vi "Acquisition Message Loop.vi"(8 "error in (no error)":errorcluster, 9 "Data Queue":refnum<queue>, 10 "Data Notifier":refnum<notifier>, 11 "Message Queues":T1) -> (0 "error out":errorcluster)   [LabVIEW 2013, in "Acquisition.lvlib"]
doc: "Message loop for handling messages pertaining to the acquisition of data from the hardware."
uses:
  Acquisition.lvlib
  support/Message Queue/All Message Queues.ctl
  support/Message Queue/Message Cluster.ctl
  Hardware Configuration.ctl
  Signal Type.ctl
  Acquisition State.ctl
  controls/UI Data.ctl
  <vilib>/Utility/error.llb/DialogType.ctl
  <vilib>/Utility/error.llb/Error Cluster From Error Code.vi
  support/Message Queue/Enqueue Message (Single).vi
  <vilib>/ErrorRing/Error Ring.xnode
  support/Message Queue/Message Queue.lvlib
  support/Message Queue/Enqueue Message (MultiLine String w Array).vi
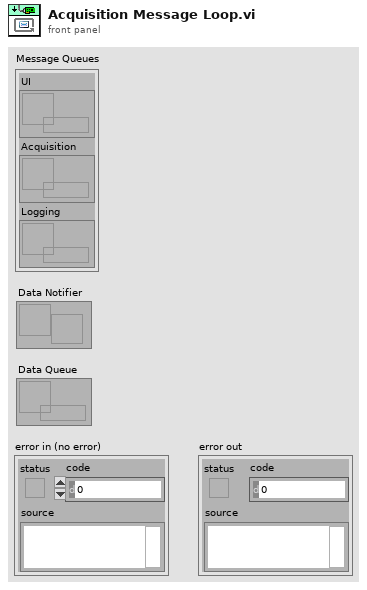
[diagram p1: front panel]
types:
  T1 = typedef "Message Queue.lvlib/All Message Queues.ctl" = cluster{"UI":refnum<queue>, "Acquisition":refnum<queue>, "Logging":refnum<queue>}
  T2 = cluster{"Macro:Initialize":string, "Macro:Exit":string, "Core":cluster{"Current VI Reference":refnum<vi>, "Close Panel on Exit?":bool}}
  T3 = typedef "UI Data.ctl" = cluster{"Start Ref":refnum<vi>, "Stop Ref":refnum<vi>, "Settings Ref":refnum<vi>, "Exit Ref":refnum<vi>, "Status Ref":refnum<vi>, "Data Ref":refnum<vi>}
  T4 = typedef "Acquisition.lvlib/Acquisition State.ctl" = enum16{"Idle", "Acquiring"}
  T5 = typedef "Acquisition.lvlib/Hardware Configuration.ctl" = cluster{"HW Refnum <Replace Me>":string, "Signal Type <Replace Me>":T6}
  T6 = typedef "Acquisition.lvlib/Signal Type.ctl" = enum16{"Sine Wave", "Square with Noise"}
  T7 = enum32{"invalid app kind", "Development System", "Run Time System", "Student Edition", "Embedded LabVIEW", "Evaluation", "Custom"}
  T8 = enum32{"Invalid", "Standard", "Closed", "Hidden", "Minimized", "Maximized"}
  T9 = typedef "DialogType.ctl" = u16
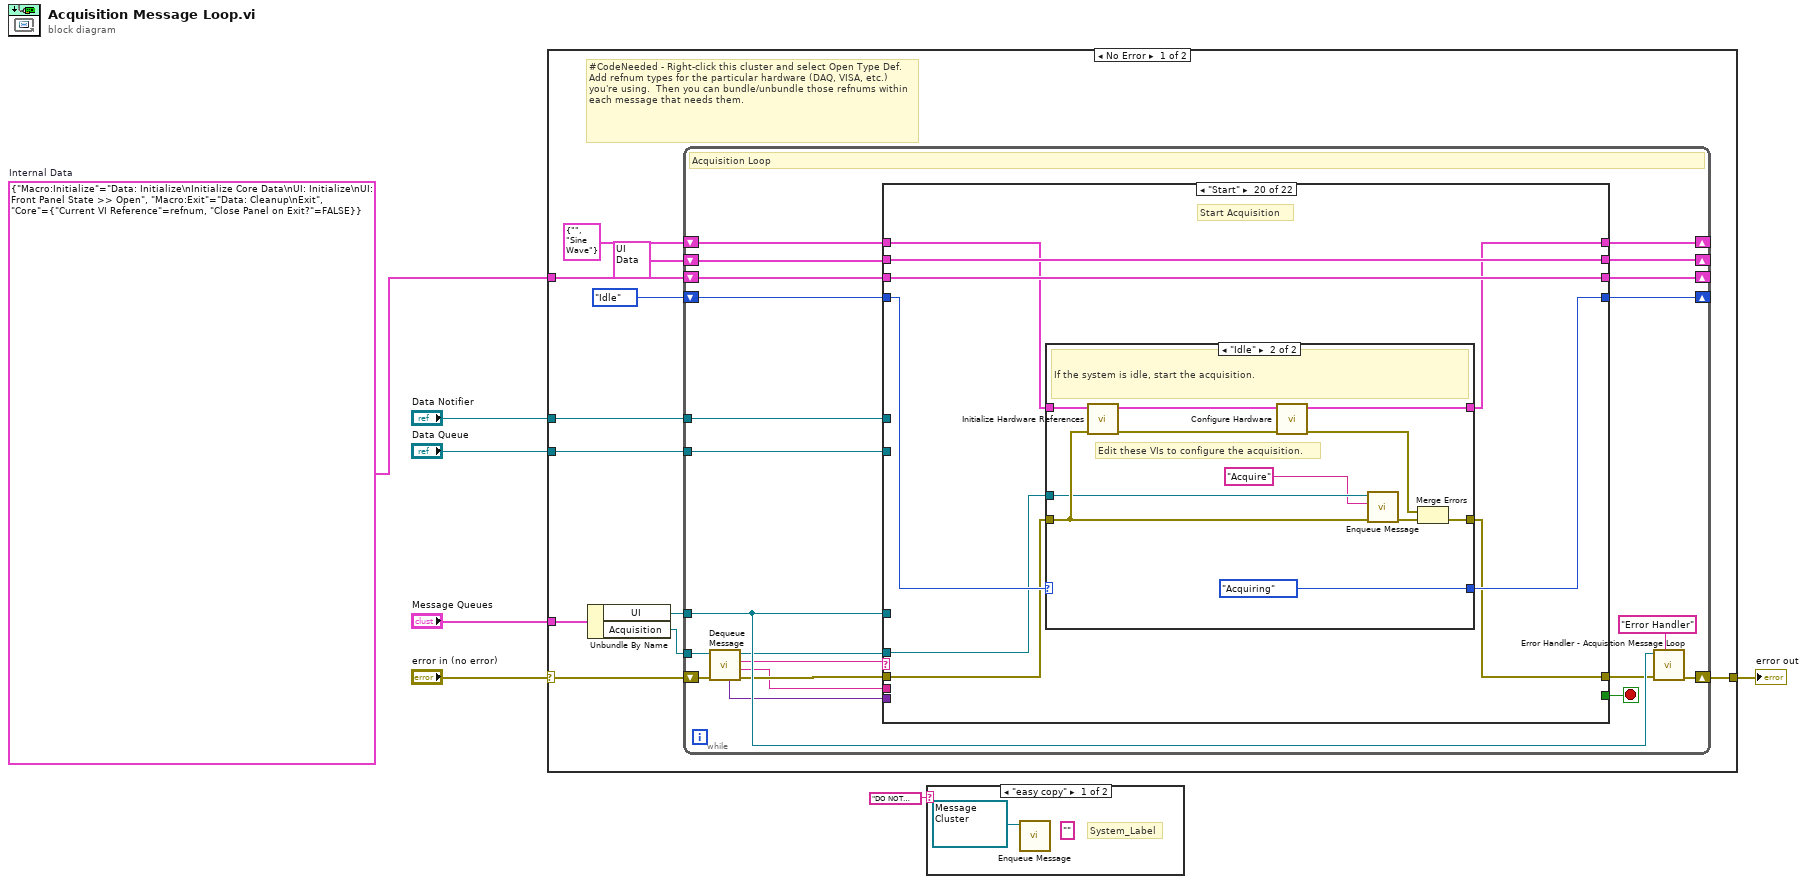
[diagram p0: block diagram]
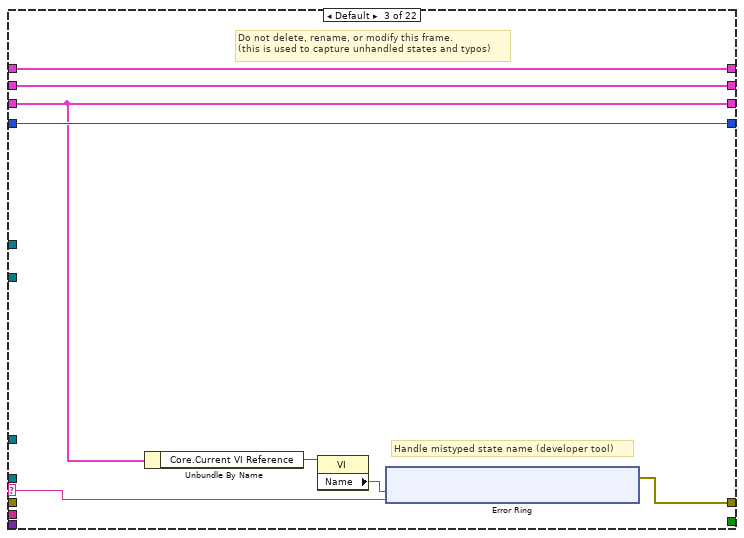
[diagram p5: hidden frame]
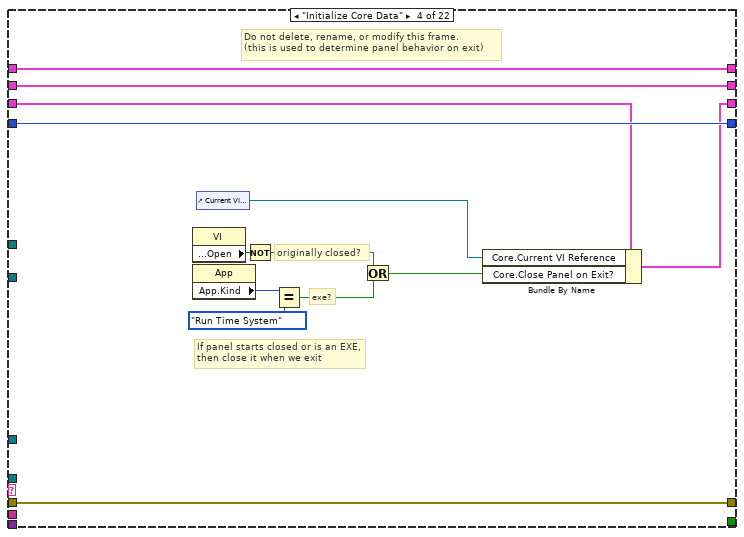
[diagram p6: hidden frame]
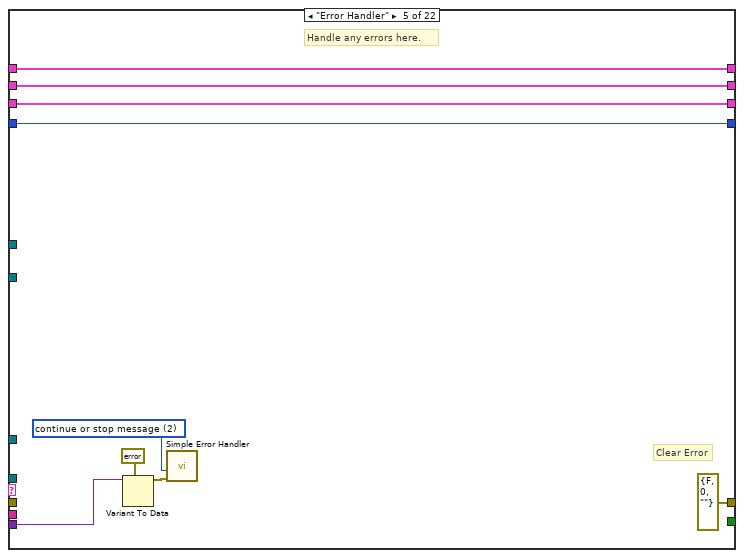
[diagram p7: hidden frame]
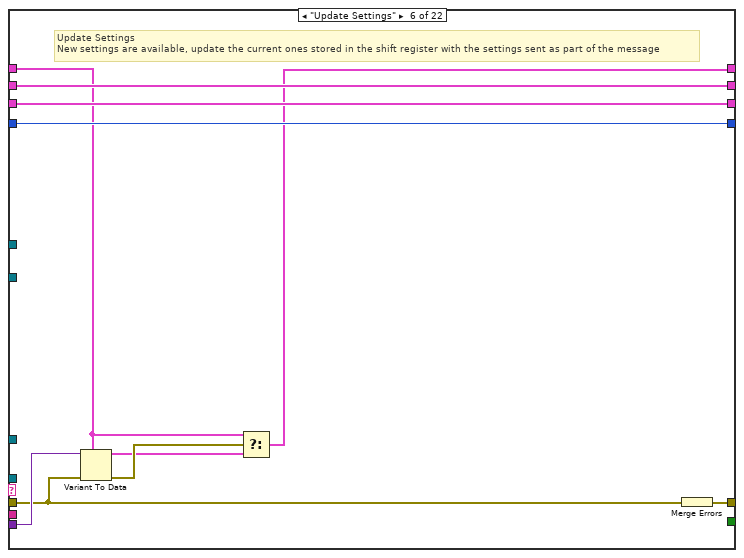
[diagram p8: hidden frame]
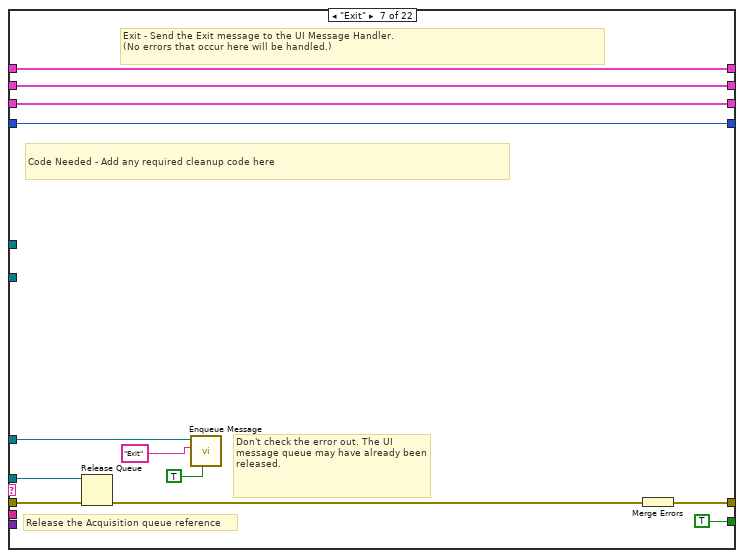
[diagram p9: hidden frame]
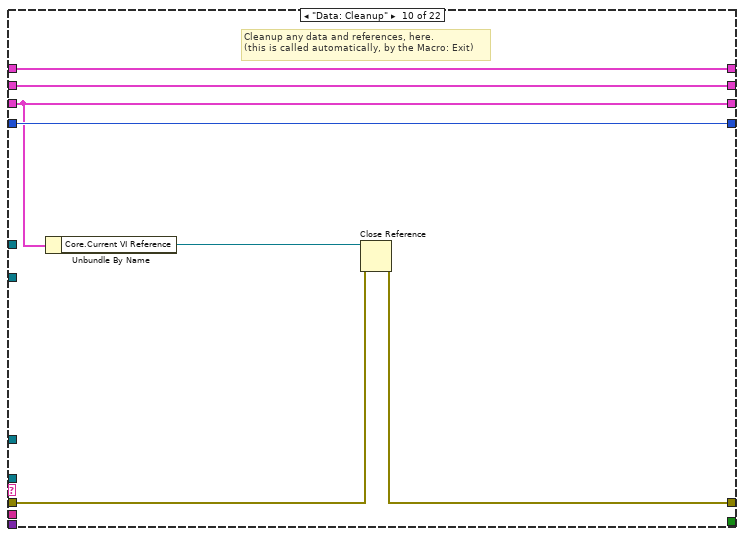
[diagram p12: hidden frame]
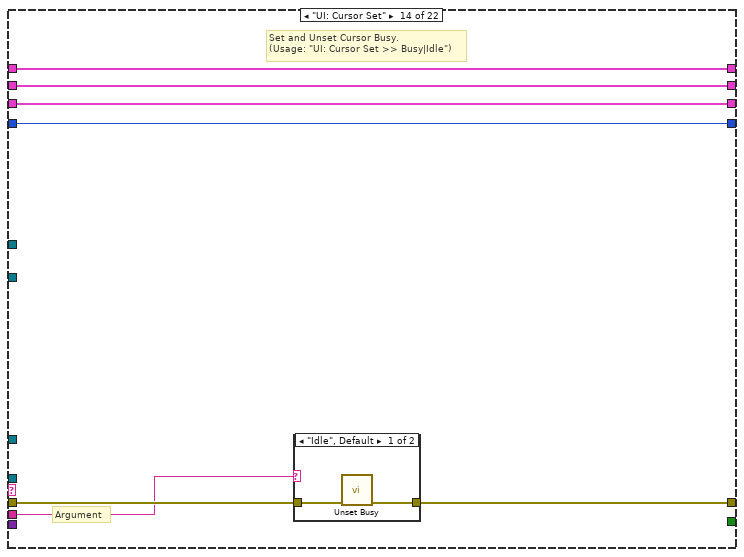
[diagram p16: hidden frame]
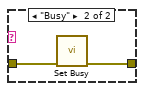
[diagram p17: hidden frame]
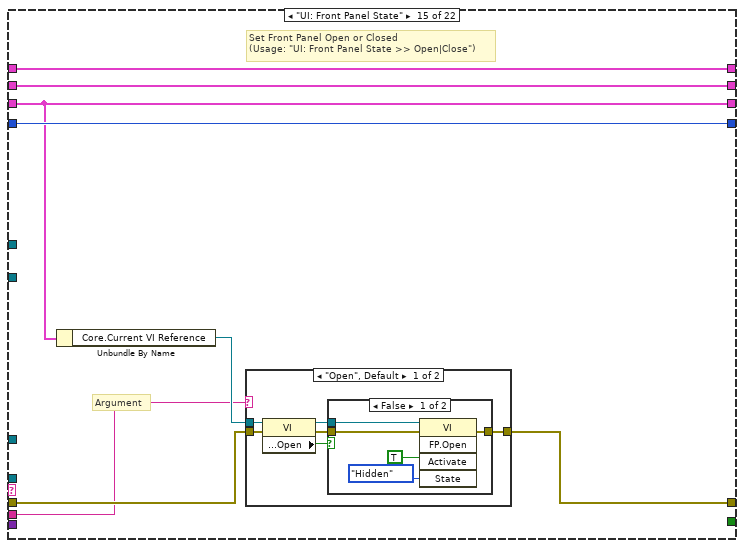
[diagram p18: hidden frame]
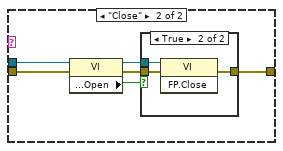
[diagram p20: hidden frame]
diagram:
  w2 = T2 {"Macro:Initialize"="Data: Initialize\nInitialize Core Data\nUI: Initialize\nUI: Front Panel State >> Open", "Macro:Exit"="Data: Cleanup\nExit", "Core"={"Current VI Reference"=refnum, "Close Panel on Exit?"=FALSE}}  # Internal Data
  n1 = case shown="No Error" "error in (no error)" {
    selector: "error in (no error)" -> [w14 w284]
    tunnel: "Message Queues" -> [w18 _]
    tunnel: [w16 w284] -> w6
    tunnel: "Data Notifier" -> [w12 _]
    tunnel: "Data Queue" -> [w11 _]
    tunnel: w2 -> [w9 _]
    frame No Error {
      # "#CodeNeeded - Right-click this cluster and select Open Type Def.  Add refnum types for the particular hardware (DAQ, VISA, etc.) you're using.  Then you can bundle/unbundle those refnums within each message that needs them."
      n2 = Unbundle By Name(w18) -> ("UI"=w13:refnum<queue>, "Acquisition"=w17:refnum<queue>)
      n3 = while {
        tunnel: w17 -> [w39]
        shift-right: [w22] -> _
        shift-left: T5 {"HW Refnum <Replace Me>"="", "Signal Type <Replace Me>"=enum."Sine Wave"} ("Data Cluster") -> [w29]
        shift-right: [w38] -> w16
        shift-left: w14 -> [w40]
        tunnel: w13 -> [w37]
        tunnel: w12 -> [w21]
        tunnel: w11 -> [w20]
        shift-right: [w23] -> _
        shift-left: Acquisition_State."Idle" ("State") -> [w27]
        shift-right: [w25] -> _
        shift-left: T3 {"Start Ref"=refnum, "Stop Ref"=refnum, "Settings Ref"=refnum, "Exit Ref"=refnum, "Status Ref"=refnum, "Data Ref"=refnum} ("Measurement UI Controls") -> [w26]
        shift-right: [w24] -> _
        shift-left: w9 -> [w28]
        stop <- w36 stop-if-true
        # "Acquisition Loop"
        n4 = call "Dequeue Message.vi"("error in (no error)"=w40, "Message Queue"=w39) -> ("error out"=w32:errorcluster, "Argument"=w31:string, "Message"=w33:string, "dup Message Queue"=w34:refnum<queue>, "Message Data"=w30:variant)  [unwired: 5 in]
        n5 = case shown="\"Start\"" w33 {
          selector: w33 -> [_ _ w53 _ _ _ _ _ _ _ _ _ _ _ _ _ _ _ _ _ w241 _]
          tunnel: w26 -> [w44 w48 w57 w71 w88 w98 w108 w113 w120 w123 w130 w135 w140 w145 w156 w186 w195 w209 w215 w226 w252 w274]
          tunnel: w31 -> [_ _ _ _ _ _ _ _ _ _ _ _ _ w146 w157 _ _ _ _ _ _ _]
          tunnel: w29 -> [w43 w49 w58 w69 w86 w92 w110 w114 w116 w124 w131 w137 w142 w149 w159 w187 w196 w207 w216 w219 w250 w268]
          tunnel: [w45 w50 w51 w79 errorcluster {"status"=FALSE, "code"=0, "source"=""} ("error out") w90 w100 w115 w117 w125 w132 w136 w141 w147 w160 w188 w191 w197 w217 w221 w242 w267] -> w35
          tunnel: w32 -> [w45 w50 _ w79 _ w89 w105 w115 w117 w126 w132 w136 w141 w148 w161 w188 w193 w206 w217 w222 w243 w270]
          tunnel: [w44 w48 w57 w71 w88 w98 w108 w113 w120 w123 w130 w135 w140 w145 w156 w186 w195 w209 w215 w226 w252 w274] -> w25
          tunnel: [_ _ _ _ _ _ TRUE _ _ _ _ _ _ _ _ _ _ _ _ _ _ _] -> w36
          tunnel: [w43 w49 w58 w69 w86 w91 w110 w114 w116 w124 w131 w137 w142 w149 w159 w187 w196 w207 w216 w218 w249 w268] -> w22
          tunnel: [w42 w47 w56 w70 w87 w97 w107 w112 w119 w122 w129 w134 w139 w144 w155 w185 w194 w208 w214 w223 w247 w271] -> w23
          tunnel: w27 -> [w42 w47 w56 w70 w87 w97 w107 w112 w119 w122 w129 w134 w139 w144 w155 w185 w194 w208 w214 w224 w248 w272]
          tunnel: w30 -> [_ _ _ _ w82 w95 _ _ _ _ _ _ _ _ _ _ _ _ _ _ _ _]
          tunnel: w28 -> [w41 w46 w52 w68 w85 w96 w106 w111 w118 w121 w128 w133 w138 w143 w154 w184 w189 w200 w213 w225 w251 w273]
          tunnel: [w41 w46 w52 w67 w85 w96 w106 w111 w118 w121 w128 w133 w138 w143 w154 w184 w189 w200 w213 w225 w251 w273] -> w24
          tunnel: w34 -> [_ _ _ _ _ _ w104 _ _ _ _ _ _ _ _ _ w192 w205 _ w220 w244 _]
          tunnel: w37 -> [_ _ _ _ _ _ w103 _ _ _ _ _ _ _ _ _ _ _ _ _ _ w269]
          tunnel: w21 -> [_ _ _ _ _ _ _ _ _ _ _ _ _ _ _ _ _ _ _ _ w246 _]
          tunnel: w20 -> [_ _ _ _ _ _ _ _ _ _ _ _ _ _ _ _ _ _ _ _ w245 _]
          frame "", "Idle" {
            # "Executes when the state queue is empty\nAlso commented out messages"
          }
          frame "---------- Core ----------" {
            # "Do not put any code in this frame.\n(it is a separator no-op)"
          }
          frame Default {
            # "Handle mistyped state name (developer tool)"
            # "Do not delete, rename, or modify this frame.\n(this is used to capture unhandled states and typos)"
            n6 = Unbundle By Name(w52) -> ("Core.Current VI Reference"=w54:refnum<vi>)
            n7 = property class="VI"(reference=w54) -> ("Name"=w55:string)  [unwired: 1 in, 2 out]
            n8 = xnode "Error Ring"("parameter 0"=w55, "parameter 1"=w53) -> ("error out"=w51:errorcluster)
          }
          frame "Initialize Core Data" {
            # "Do not delete, rename, or modify this frame.\n(this is used to determine panel behavior on exit)"
            # "originally closed?"
            # "exe?"
            # "If panel starts closed or is an EXE, then close it when we exit"
            n9 = property class="VI"() -> ("Front Panel.Open"=w78:bool)  [unwired: 2 in, 2 out]
            n10 = property class="App"() -> ("App.Kind"=w77:T7)  [unwired: 2 in, 2 out]
            n11 = control-ref of="Current VI Reference"() -> (w72:refnum<vi>)
            n12 = Not(x=w78) -> (.not. x?=w75:bool)
            n13 = Equal?(x=w77, y=T7."Run Time System" ("Application:Kind")) -> (x = y?=w74:bool)
            n14 = Or(x=w75, y=w74) -> (x .or. y?=w73:bool)
            n15 = Bundle By Name(cluster=w68, "Core.Current VI Reference"=w72, "Core.Close Panel on Exit?"=w73) -> (w67:T2)
          }
          frame "Error Handler" {
            w81 = T9 2 items=["no dialog", "OK message", "continue or stop message", "OK message + warnings", "continue/stop + warnings"] ("type of dialog (OK msg:1)")
            # "Clear Error"
            # "Handle any errors here."
            n16 = Variant To Data(type=errorcluster {"status"=FALSE, "code"=0, "source"=""} ("error constant"), Variant=w82) -> (data=w84:errorcluster)  [unwired: 1 in, 1 out]
            n17 = call <vilib>:"Simple Error Handler.vi"("type of dialog (OK msg:1)"=w81, "error in (no error)"=w84) -> ()  [unwired: 3 in, 5 out]
          }
          frame "Update Settings" {
            # "Update Settings\nNew settings are available, update the current ones stored in the shift register with the settings sent as part of the message"
            n18 = Variant To Data(error in=w89, type=w92, Variant=w95) -> (data=w93:T5, error out=w94:errorcluster)
            n19 = Select(t=w92, s=w94, f=w93) -> (s? t:f=w91:T5)
            n20 = Merge Errors(w89) -> (w90:errorcluster)
          }
          frame "Exit" {
            # "Code Needed - Add any required cleanup code here"
            # "Exit - Send the Exit message to the UI Message Handler.\n(No errors that occur here will be handled.)"
            # "Don't check the error out. The UI message queue may have already been released."
            # "Release the Acquisition queue reference"
            n21 = Release Queue(queue=w104, error in (no error)=w105) -> (error out=w99:errorcluster)  [unwired: 1 in, 2 out]
            n22 = call-poly "Enqueue Message.vi"("Priority Message? (F)"=TRUE, "Message"="Exit", "Message Queue"=w103) -> ()  [unwired: 7 in, 2 out]
            n23 = Merge Errors(w99) -> (w100:errorcluster)
          }
          frame "---------- Data ----------" {
            # "Do not put any code in this frame.\n(It is a separator no-op. You can make a copy of this frame to create a new Data frame)"
          }
          frame "Data: Initialize" {
            # "nothing right now"
            # "Initialize the shift-register data, here.\n(data names are defined by what you wire into the bundle function)"
          }
          frame "Data: Cleanup" {
            # "Cleanup any data and references, here.\n(this is called automatically, by the Macro: Exit)"
            n24 = Unbundle By Name(w121) -> ("Core.Current VI Reference"=w127:refnum<vi>)
            n25 = Close Reference(reference=w127, error in (no error)=w126) -> (error out=w125:errorcluster)
          }
          frame "---------- UI ----------" {
            # "Do not put any code in this frame.\n(It is a separator no-op. You can make a copy of this frame to create a new UI frame)"
          }
          frame "UI: Initialize" {
            # "Initialize the User Interface, here.\n(this is called automatically, by the Macro: Init)"
          }
          frame "UI: Initialize UI Refs" {
            # "Package and Init UI Refs as Required"
          }
          frame "UI: Cursor Set" {
            # "Argument"
            # "Set and Unset Cursor Busy.\n(Usage: \"UI: Cursor Set >> Busy|Idle\")"
            n26 = case shown="\"Idle\", Default" w146 {
              tunnel: w148 -> [w151 w153]
              tunnel: [w150 w152] -> w147
              frame "Idle", Default {
                n27 = call <vilib>:"Unset Busy.vi"("error in (no error)"=w151) -> ("error out"=w150:errorcluster)  [unwired: 10 in]
              }
              frame "Busy" {
                n28 = call <vilib>:"Set Busy.vi"("error in (no error)"=w153) -> ("error out"=w152:errorcluster)  [unwired: 9 in, 1 out]
              }
            }
          }
          frame "UI: Front Panel State" {
            # "Argument"
            # "Set Front Panel Open or Closed\n(Usage: \"UI: Front Panel State >> Open|Close\")"
            n29 = Unbundle By Name(w154) -> ("Core.Current VI Reference"=w158:refnum<vi>)
            n30 = case shown="\"Open\", Default" w157 {
              tunnel: w161 -> [w165 w178]
              tunnel: [w167 w179] -> w160
              tunnel: w158 -> [w166 w176]
              frame "Open", Default {
                n31 = property class="VI"(reference=w166, error in=w165) -> (reference out=w163:refnum<vi>, error out=w164:errorcluster, "Front Panel.Open"=w162:bool)
                n32 = case shown="False" w162 {
                  tunnel: [w170 w173] -> w167
                  tunnel: w164 -> [w169 w173]
                  tunnel: w163 -> [w168 _]
                  frame False {
                    n33 = invoke class="VI" method="FP.Open"(reference=w168, error in=w169, "Activate"=TRUE, "State"=T8."Hidden") -> (error out=w170:errorcluster)  [unwired: 1 in, 4 out]
                  }
                  frame True {
                  }
                }
              }
              frame "Close" {
                n34 = property class="VI"(reference=w176, error in=w178) -> (reference out=w175:refnum<vi>, error out=w177:errorcluster, "Front Panel.Open"=w174:bool)
                n35 = case shown="True" w174 {
                  tunnel: [w180 w183] -> w179
                  tunnel: w177 -> [w180 w182]
                  tunnel: w175 -> [_ w181]
                  frame False {
                  }
                  frame True {
                    n36 = invoke class="VI" method="FP.Close"(reference=w181, error in=w182) -> (error out=w183:errorcluster)  [unwired: 1 in, 2 out]
                  }
                }
              }
            }
          }
          frame "---------- Macro ----------" {
            # "Do not put any code in this frame.\n(It is a separator no-op. You can make a copy of this frame to create a new Macro frame)"
          }
          frame "Macro: Initialize" {
            # "Initialization Macro\n(This is called once, when the VI starts)"
            n37 = Unbundle By Name(w189) -> ("Macro:Initialize"=w190:string)
            n38 = call-poly "Enqueue Message.vi"("error in (no error)"=w193, "Message"=w190, "Message Queue"=w192) -> ("error out"=w191:errorcluster)  [unwired: 7 in, 1 out]
          }
          frame "Macro: Exit" {
            # "Exit Macro\n(This is called once, when the VI exits)"
            n39 = Unbundle By Name(w200) -> ("Core.Close Panel on Exit?"=w212:bool)
            n40 = Unbundle By Name(w200) -> ("Macro:Exit"=w199:string)
            n41 = Select(t="UI: Front Panel State >> Close", s=w212, f="") -> (s? t:f=w204:string)
            n42 = call-poly "Enqueue Message.vi"("Priority Message? (F)"=TRUE, "error in (no error)"=w206, "Message"=w204, "Message Queue"=w205) -> ("error out"=w201:errorcluster, "dup Message Queue"=w202:refnum<queue>)  [unwired: 6 in]
            n43 = call-poly "Enqueue Message.vi"("Priority Message? (F)"=FALSE, "error in (no error)"=w201, "Message"=w199, "Message Queue"=w202) -> ("error out"=w197:errorcluster)  [unwired: 6 in, 1 out]
          }
          frame "---------- Acquisition ----------" {
            # "Acquisition Section"
          }
          frame "Start" {
            # "Start Acquisition"
            n44 = case shown="\"Idle\"" w224 {
              selector: w224 -> [w227 _]
              tunnel: [w228 w240] -> w221
              tunnel: w219 -> [w229 w239]
              tunnel: w222 -> [w228 w238]
              tunnel: w220 -> [_ w236]
              tunnel: [w229 w232] -> w218
              tunnel: [w227 Acquisition_State."Acquiring" ("Acquisition State")] -> w223
              frame "Acquiring" {
                # "The system is already acquiring. Ignore the \"Start\" message."
              }
              frame "Idle" {
                # "Edit these VIs to configure the acquisition."
                # "If the system is idle, start the acquisition."
                n45 = call "Initialize Hardware References.vi"("error in (no error)"=w238, "Hardware Resources in"=w239) -> ("error out"=w235:errorcluster, "Hardware Resources out"=w233:T5)  [unwired: 8 in]
                n46 = call "Configure Hardware.vi"("error in (no error)"=w235, "Hardware Resources in"=w233) -> ("error out"=w234:errorcluster, "Hardware Resources out"=w232:T5)  [unwired: 8 in]
                n47 = call-poly "Enqueue Message.vi"("error in (no error)"=w238, "Message"="Acquire", "Message Queue"=w236) -> ("error out"=w237:errorcluster)  [unwired: 7 in, 1 out]
                n48 = Merge Errors(w234, w237) -> (w240:errorcluster)
              }
            }
          }
          frame "Acquire" {
            # "Acquire Data"
            n49 = case shown="\"Acquiring\"" w248 {
              selector: w248 -> [w253 w258]
              tunnel: [w254 w266] -> w242
              tunnel: w244 -> [_ w264]
              tunnel: w243 -> [w254 w257]
              tunnel: [w255 w262] -> w249
              tunnel: w250 -> [w255 w261]
              tunnel: w246 -> [_ w260]
              tunnel: w245 -> [_ w259]
              tunnel: [w253 w258] -> w247
              tunnel: w241 -> [_ w256]
              frame "Idle" {
                # "Ignore \"Acquire\" messages when the acquisition is idle."
              }
              frame "Acquiring" {
                # "Acquire more data while in the \"Acquiring\" state."
                n50 = call "Acquire.vi"("error in (no error)"=w257, "Data Queue"=w259, "Data Notifier"=w260, "Hardware Resources in"=w261) -> ("error out"=w263:errorcluster, "Hardware Resources out"=w262:T5)  [unwired: 6 in]
                n51 = call-poly "Enqueue Message.vi"("error in (no error)"=w257, "Message"=w256, "Message Queue"=w264) -> ("error out"=w265:errorcluster)  [unwired: 7 in, 1 out]
                n52 = Merge Errors(w263, w265) -> (w266:errorcluster)
              }
            }
          }
          frame "Stop" {
            # "Stop Acquiring Data"
            n53 = case shown="\"Acquiring\"" w272 {
              selector: w272 -> [w275 _]
              tunnel: w270 -> [w276 w283]
              tunnel: [w276 w279] -> w267
              tunnel: w268 -> [_ w281]
              tunnel: [w275 Acquisition_State."Idle" ("State")] -> w271
              tunnel: w269 -> [_ w278]
              frame "Idle" {
                # "The system is already idle. Ignore the \"Stop\" message."
              }
              frame "Acquiring" {
                # "If the system is acquiring, stop the acquisition."
                n54 = call "Stop Acquisition.vi"("error in (no error)"=w283, "Hardware Resources in"=w281) -> ("error out"=w282:errorcluster)  [unwired: 9 in]
                n55 = call-poly "Enqueue Message.vi"("error in (no error)"=w282, "Message"="Acquisition Stopped", "Message Queue"=w278) -> ("error out"=w279:errorcluster)  [unwired: 7 in, 1 out]
              }
            }
          }
        }
        n56 = call "Error Handler - Acquisition Message Loop.vi"("Error Handler Message"="Error Handler" ("Message"), "error in (no error)"=w35, "Message Queue"=w37) -> ("dup error in"=w38:errorcluster)  [unwired: 7 in, 1 out]
      }
    }
    frame Error {
    }
  }
  "error out" <- w6
  n57 = case shown="\"easy copy\"" "DO NOT RUN!!" {
    frame "easy copy" {
      (unwired) "" ("Message")
      # "System_Label"
      n58 = call-poly "Enqueue Message.vi"("Message Queue"=refnum<queue> refnum) -> ()  [unwired: 9 in, 2 out]
    }
    frame Default {
    }
  }
